vi "Ref_Num_Test_Conf.vi"(0 "Device Types":refnum<vi>, 1 "Test Fixtures":refnum<vi>, 2 "Test Signal Level":refnum<vi>, 4 "Device Type (OUTPUT)":refnum<vi>, 5 "Test Types":refnum<vi>, 6 "Test Fixture (OUTPUT)":refnum<vi>, 7 "Confirm Configuration":refnum<vi>, 10 "Test Type (OUTPUT)":refnum<vi>, 11 "error in":errorcluster, 12 "Category":refnum<vi>, 13 "LowCapMode?":refnum<vi>, 14 "CAPACITANCE TEST?":refnum<vi>) -> (15 "error out":errorcluster)   [LabVIEW 2020]
panel:
  in  "IGBT : Test Type":string[](array[string])
  in  "Transistor : Test Type":string[](array[string])
  in  "MOSFET : Test Type":string[](array[string])
  out "Fixture File Name":string
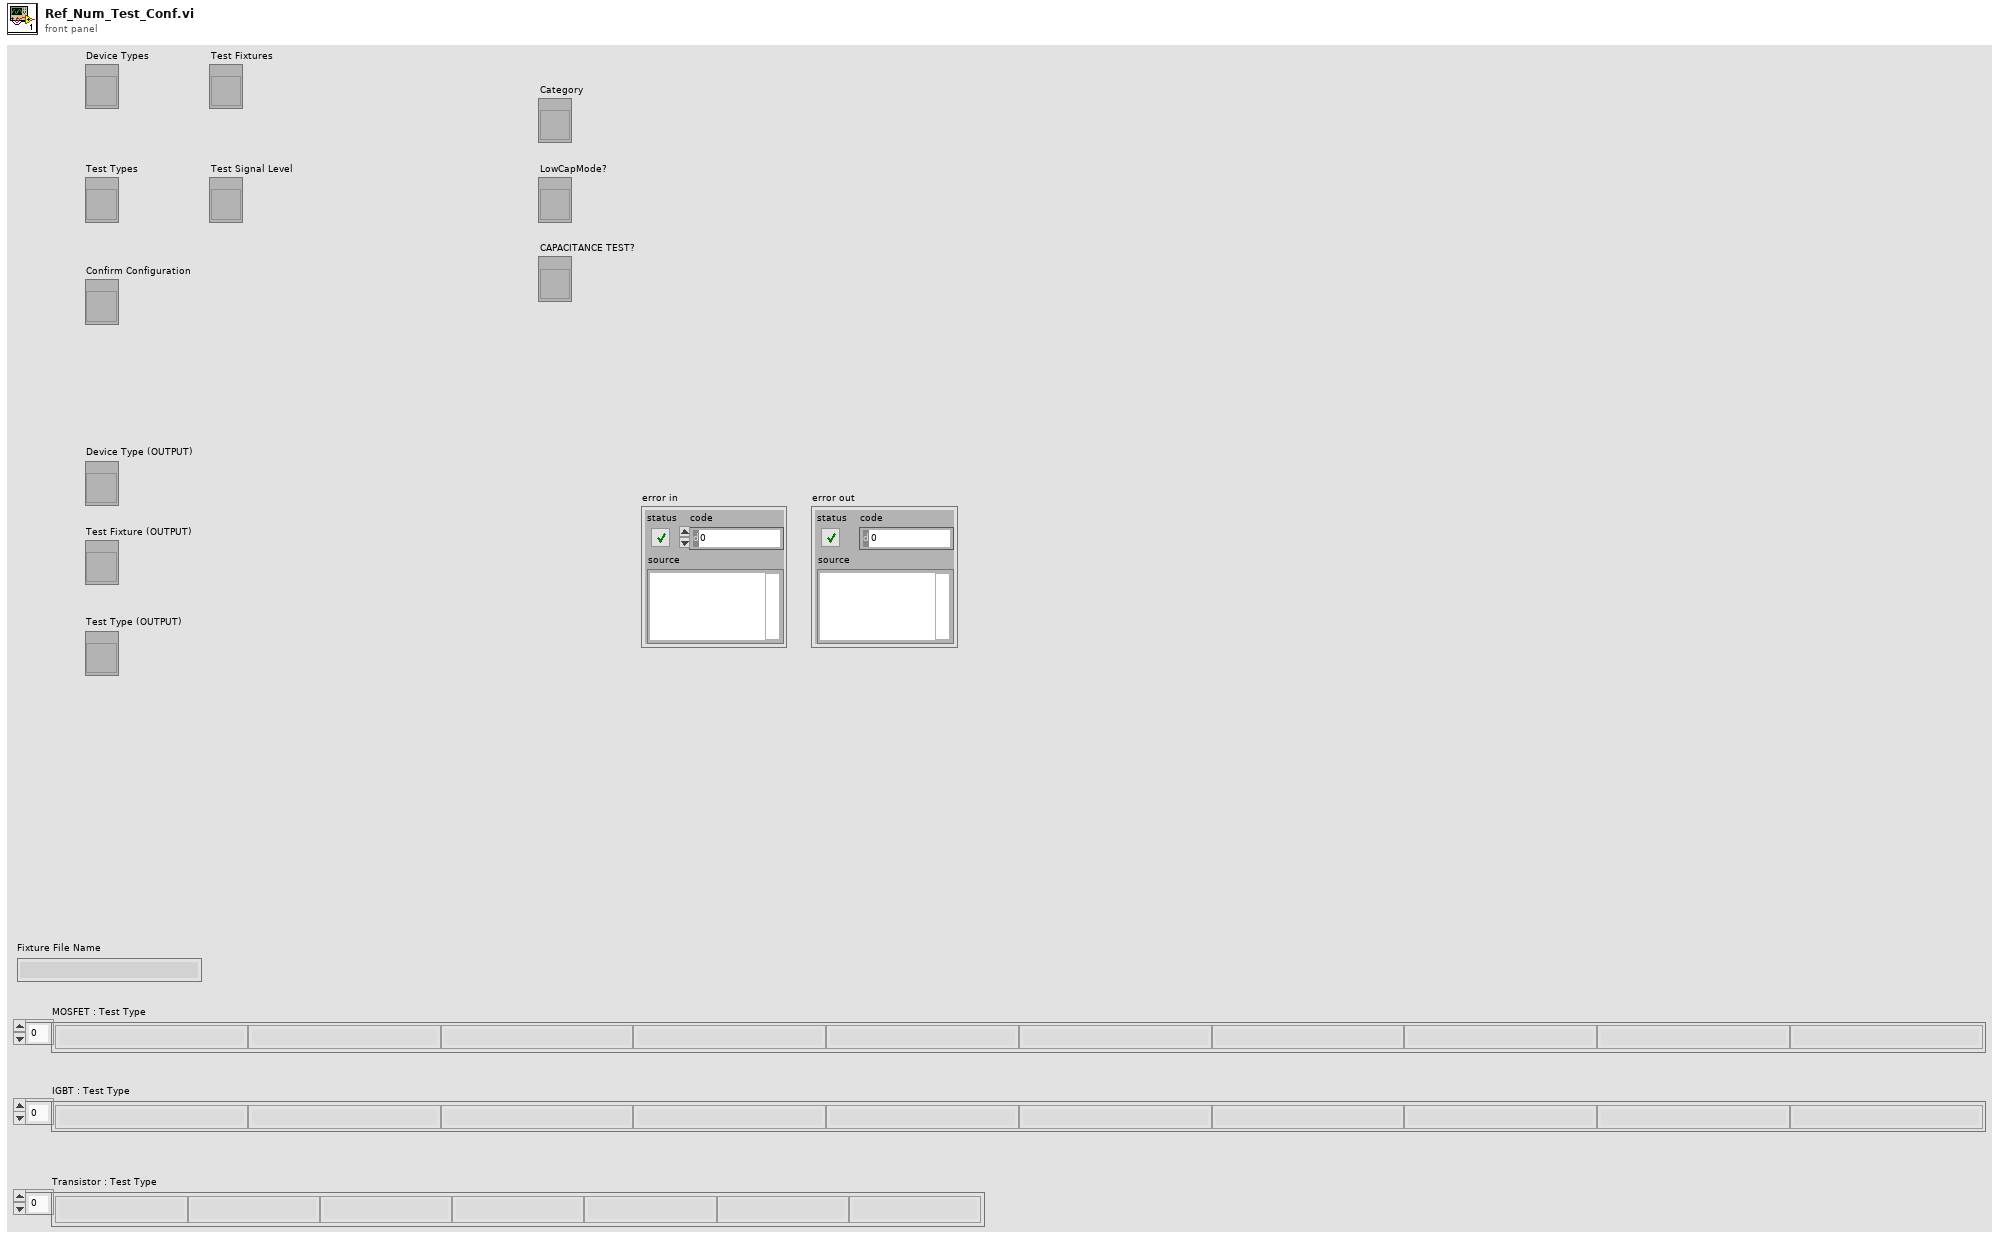
[diagram p1: front panel]
types:
  T1 = enum16{"Diode", "Transistor", "MOSFET", "Thyristor", "IGBT"}
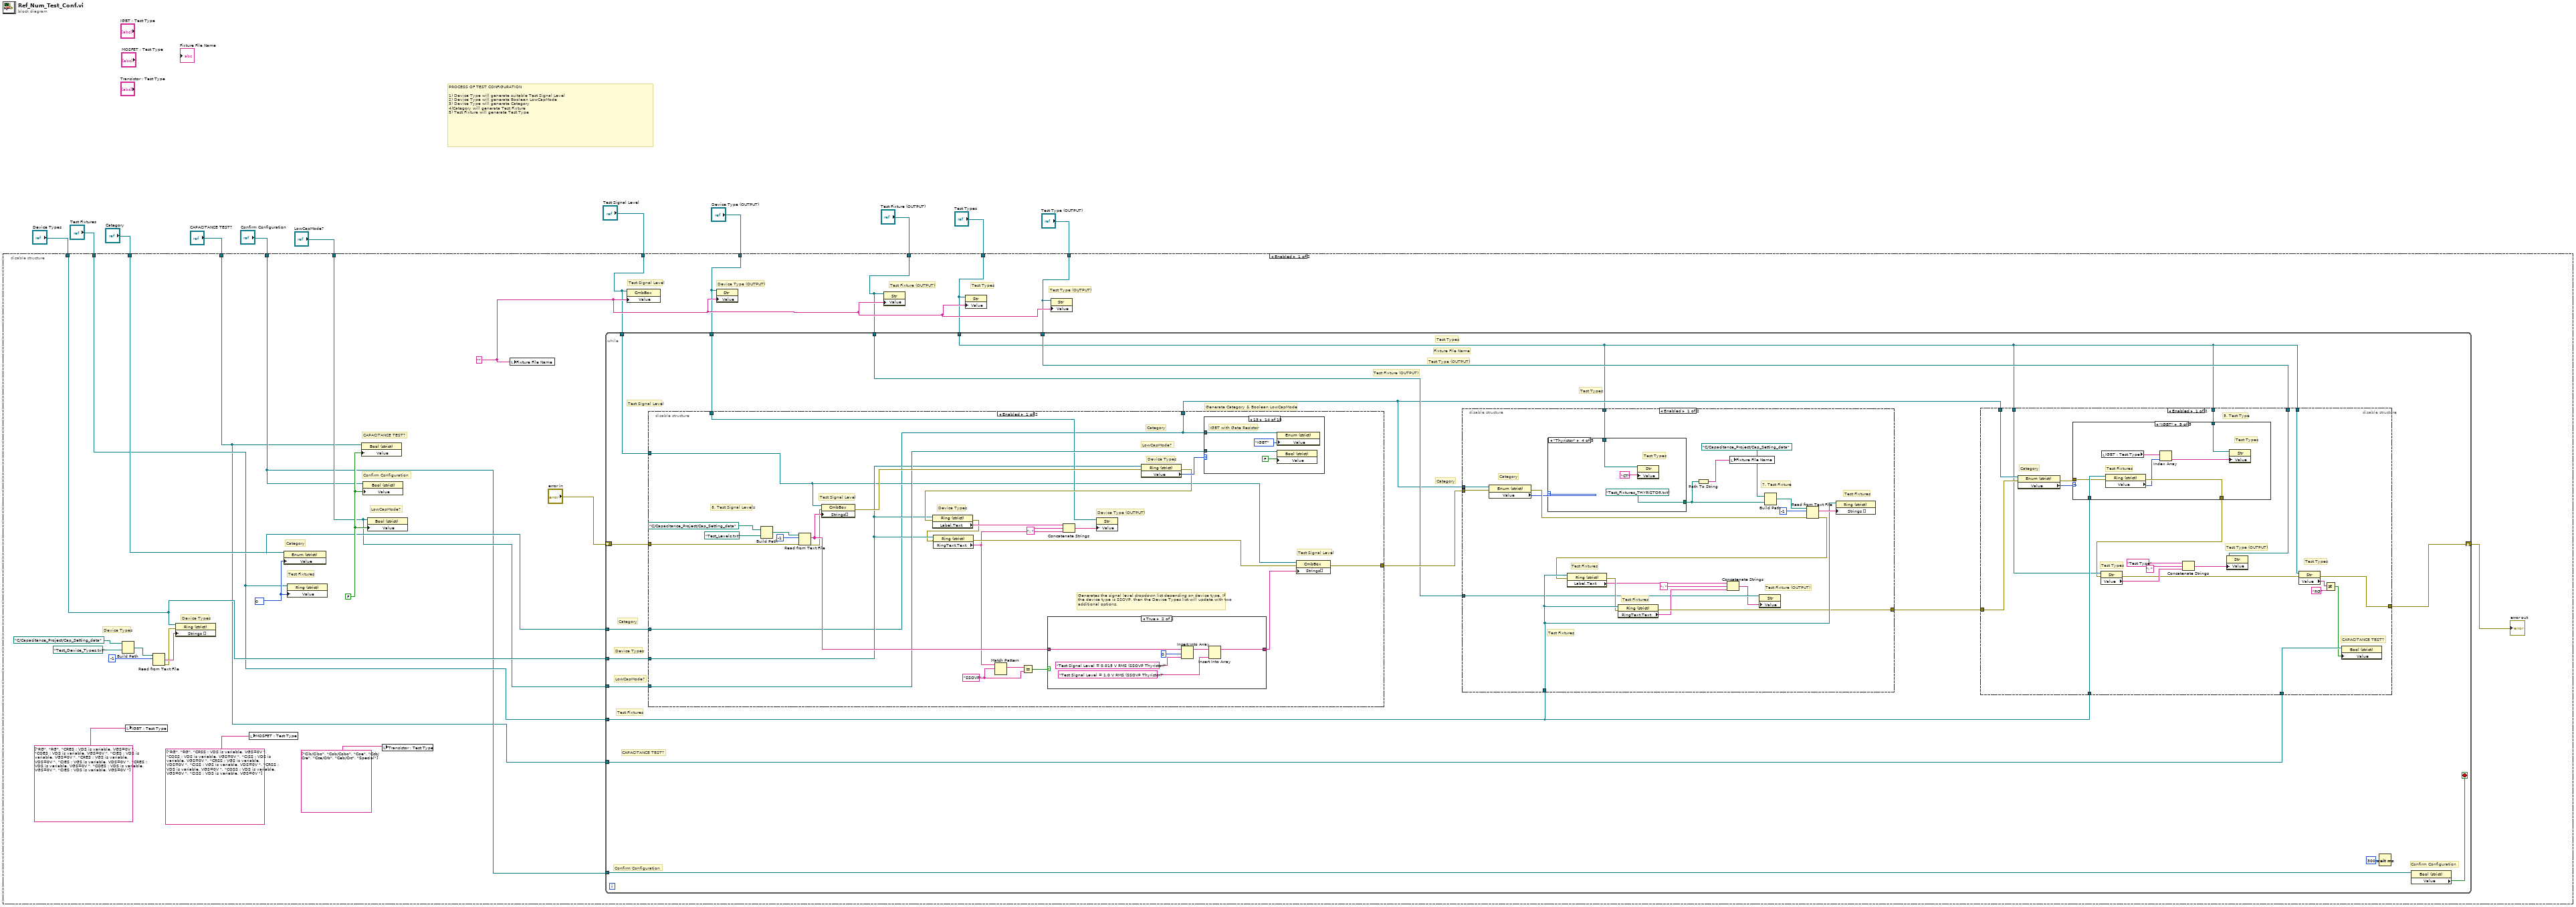
[diagram p0: block diagram]
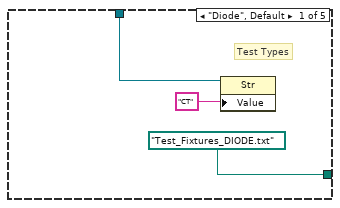
[diagram p2: hidden frame]
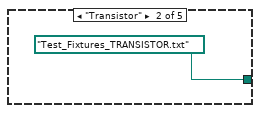
[diagram p3: hidden frame]
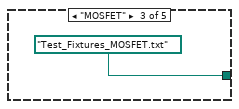
[diagram p4: hidden frame]
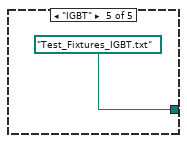
[diagram p5: hidden frame]
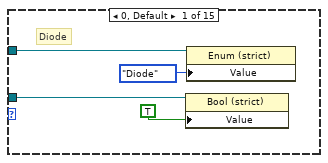
[diagram p7: hidden frame]
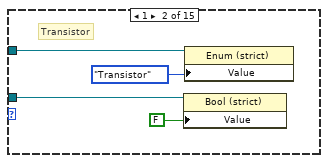
[diagram p8: hidden frame]
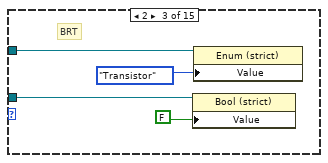
[diagram p9: hidden frame]
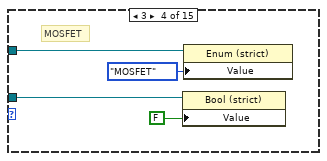
[diagram p10: hidden frame]
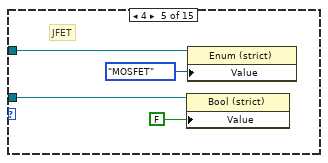
[diagram p11: hidden frame]
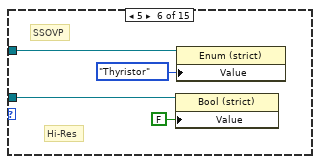
[diagram p12: hidden frame]
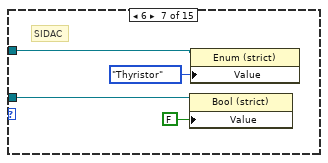
[diagram p13: hidden frame]
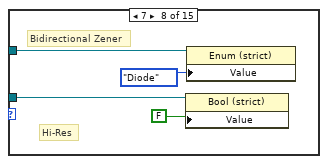
[diagram p14: hidden frame]
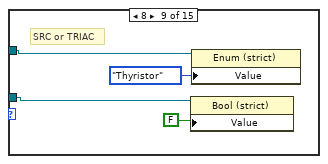
[diagram p15: hidden frame]
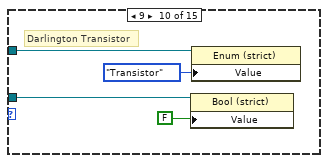
[diagram p16: hidden frame]
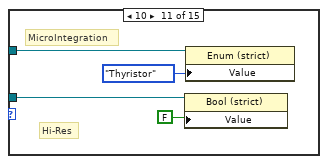
[diagram p17: hidden frame]
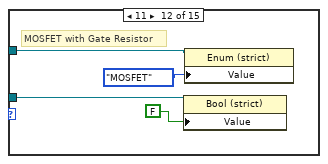
[diagram p18: hidden frame]
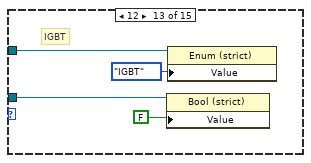
[diagram p19: hidden frame]
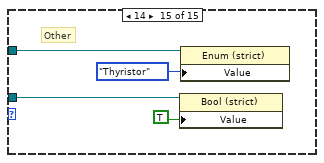
[diagram p20: hidden frame]
diagram:
  # "PROCESS OF TEST CONFIGURATION\n\n1) Device Type will generate suitable Test Signal Level\n2) Device Type will generate Boolean LowCapMode\n3) Device Type will generate Category\n4)Category will generate Test Fixture\n5) Test Fixture will generate Test Type"
  n1 = disable-structure shown="Enabled" {
    disable-tunnel: "Device Types" -> [w24 _]
    disable-tunnel: "Test Fixtures" -> [w19 _]
    disable-tunnel: "Category" -> [w23 _]
    disable-tunnel: "LowCapMode?" -> [w22 _]
    disable-tunnel: "Confirm Configuration" -> [w17 _]
    disable-tunnel: "CAPACITANCE TEST?" -> [w15 _]
    disable-tunnel: "Test Signal Level" -> [w25 _]
    disable-tunnel: "Device Type (OUTPUT)" -> [w21 _]
    disable-tunnel: "Test Fixture (OUTPUT)" -> [w18 _]
    disable-tunnel: "Test Types" -> [w20 _]
    disable-tunnel: "Test Type (OUTPUT)" -> [w16 _]
    frame Enabled {
      w28 = u16 0 items=[""]
      w27 = FALSE ("LowCapMode?")
      w26 = "" ("Category Check")
      # "Device Types"
      # "Test Type (OUTPUT)"
      # "Test Types"
      # "Test Fixture (OUTPUT)"
      # "Device Type (OUTPUT)"
      # "Test Signal Level"
      # "CAPACITANCE TEST?"
      # "Confirm Configuration"
      # "LowCapMode?"
      # "Category"
      # "Test Fixtures"
      # "Device Types"
      n2 = Build Path(base path=path "C:/Capacitance_Project/Cap_Setting_data", name or relative path=path "Test_Device_Types.txt" ("file (use dialog)")) -> (appended path=w36:path)
      n3 = local write "IGBT : Test Type"(string[] ["RG", "RG", "CRES : VDS is variable, VGS=0V ", "COES : VDS is variable, VGS=0V ", "CIES : VDS is variable, VGS=0V ", "CRES : VGS is variable, VDS=0V ", "CIES : VGS is variable, VDS=0V ", "CRES : VDS is variable, VGS=0V ", "COES : VDS is variable, VGS=0V ", "CIES : VDS is variable, VGS=0V "] ("MOSFET : Test Type")) -> ()
      n4 = Read from Text File(file (use dialog)=w36, count=-1) -> (text=w30:string[], error out=w29:errorcluster)  [unwired: 2 in, 2 out]
      n5 = property class="Ring (strict)"(reference=w24, error in=w29, "Strings []"=w30) -> ()  [unwired: 2 out]
      n6 = local write "MOSFET : Test Type"(string[] ["RG", "RG", "CRSS : VDS is variable, VGS=0V ", "COSS : VDS is variable, VGS=0V ", "CISS : VDS is variable, VGS=0V ", "CRSS : VGS is variable, VDS=0V ", "CISS : VGS is variable, VDS=0V ", "CRSS : VDS is variable, VGS=0V ", "COSS : VDS is variable, VGS=0V ", "CISS : VDS is variable, VGS=0V "] ("MOSFET : Test Type")) -> ()
      n7 = property class="Enum (strict)"(reference=w23, "Value"=w28) -> ()  [unwired: 1 in, 2 out]
      n8 = property class="Ring (strict)"(reference=w19, "Value"=w28) -> ()  [unwired: 1 in, 2 out]
      n9 = property class="Bool (strict)"(reference=w15, "Value"=w27) -> ()  [unwired: 1 in, 2 out]
      n10 = property class="Bool (strict)"(reference=w17, "Value"=w27) -> ()  [unwired: 1 in, 2 out]
      n11 = property class="Bool (strict)"(reference=w22, "Value"=w27) -> ()  [unwired: 1 in, 2 out]
      n12 = local write "Transistor : Test Type"(string[] ["Cib/Cibo", "Cob/Cobo", "Coe", "Ccb/Cre", "Cce/Crb", "Ceb/Crc", "Special"] ("IGBT : Test Type")) -> ()
      n13 = local write "Fixture File Name"(w26) -> ()
      n14 = while {
        shift-right: [w54] -> w14
        shift-left: "error in" -> [w53]
        tunnel: w25 -> [w50]
        tunnel: w24 -> [w49]
        tunnel: w23 -> [w48]
        tunnel: w22 -> [w47]
        tunnel: w21 -> [w46]
        tunnel: w20 -> [w38]
        tunnel: w19 -> [w40]
        tunnel: w18 -> [w44]
        tunnel: w17 -> [w42]
        tunnel: w16 -> [w39]
        tunnel: w15 -> [w37]
        stop <- w41 stop-if-true
        # "CAPACITANCE TEST?"
        # "Test Type (OUTPUT)"
        # "Confirm Configuration"
        # "Confirm Configuration"
        # "Category"
        # "Test Fixture (OUTPUT)"
        # "Test Fixtures"
        # "Fixture File Name"
        # "Test Types"
        # "Test Types"
        # "LowCapMode?"
        # "Generate Category & Boolean LowCapMode"
        # "Category"
        # "Device Types"
        # "Test Signal Level"
        n15 = disable-structure shown="Enabled" {
          disable-tunnel: [w88 _] -> w45
          disable-tunnel: w53 -> [w103 _]
          disable-tunnel: w50 -> [w91 _]
          disable-tunnel: w49 -> [w92 _]
          disable-tunnel: w48 -> [w85 _]
          disable-tunnel: w47 -> [w98 _]
          disable-tunnel: w46 -> [w94 _]
          disable-tunnel: [w85 _] -> w43
          frame Enabled {
            w108 = "SSOVP" ("regular expression")
            # "Test Signal Level"
            # "Device Type (OUTPUT)"
            # "Category"
            # "LowCapMode?"
            # "Device Types"
            # "Device Types"
            # "Test Signal Level"
            # "8. Test Signal Levels"
            # "Generates the signal level dropdown list depending on device type. If\nthe device type is SSOVP, then the Device Types list will update with two\nadditional options."
            n16 = Build Path(base path=path "C:/Capacitance_Project/Cap_Setting_data", name or relative path=path "Test_Levels.txt") -> (appended path=w106:path)
            n17 = Read from Text File(file (use dialog)=w106, count=-1, error in=w103) -> (text=w102:string[], error out=w101:errorcluster)  [unwired: 1 in, 2 out]
            n18 = property class="CmbBox"(reference=w91, error in=w101, "Strings[]"=w102) -> (error out=w100:errorcluster)  [unwired: 1 out]
            n19 = property class="Ring (strict)"(reference=w92, error in=w100) -> (error out=w97:errorcluster, "Value"=w99:u16)  [unwired: 1 out]
            n20 = property class="Ring (strict)"(reference=w92, error in=w97) -> (error out=w89:errorcluster, "Label.Text"=w95:string)  [unwired: 1 out]
            n21 = property class="Ring (strict)"(reference=w92, error in=w89) -> (error out=w90:errorcluster, "RingText.Text"=w86:string)  [unwired: 1 out]
            n22 = Match Pattern(string=w86, regular expression=w108) -> (match substring=w109:string)  [unwired: 1 in, 3 out]
            n23 = Equal?(x=w109, y=w108) -> (x = y?=w107:bool)
            n24 = case shown="True" w107 {
              tunnel: w102 -> [w170 w176]
              tunnel: [w170 w172] -> w87
              frame False {
              }
              frame True {
                n25 = Insert Into Array(array=w176, index=0, new element="Test Signal Level = 0.015 V RMS (SSOVP Thyristor)" ("new element/subarray")) -> (w173:string[])
                n26 = Insert Into Array(array=w173, new element="Test Signal Level = 1.0 V RMS (SSOVP Thyristor)" ("new element/subarray")) -> (w172:string[])  [unwired: 1 in]
              }
            }
            n27 = Concatenate Strings(w95, ": " ("string"), w86) -> (w93:string)
            n28 = property class="Str"(reference=w94, "Value"=w93) -> ()  [unwired: 1 in, 2 out]
            n29 = case shown="13" w99 {
              tunnel: w85 -> [w113 w117 w120 w125 w128 w133 w137 w141 w145 w149 w153 w157 w161 w165 w169]
              tunnel: w98 -> [w112 w115 w121 w124 w129 w132 w136 w140 w144 w148 w152 w156 w160 w164 w168]
              frame 0, Default {
                # "Diode"
                n30 = property class="Bool (strict)"(reference=w112, "Value"=TRUE ("LowCapMode?")) -> ()  [unwired: 1 in, 2 out]
                n31 = property class="Enum (strict)"(reference=w113, "Value"=T1."Diode" ("Category")) -> ()  [unwired: 1 in, 2 out]
              }
              frame 1 {
                # "Transistor"
                n32 = property class="Bool (strict)"(reference=w115, "Value"=FALSE ("LowCapMode?")) -> ()  [unwired: 1 in, 2 out]
                n33 = property class="Enum (strict)"(reference=w117, "Value"=T1."Transistor" ("Category")) -> ()  [unwired: 1 in, 2 out]
              }
              frame 2 {
                # "BRT"
                n34 = property class="Bool (strict)"(reference=w121, "Value"=FALSE ("LowCapMode?")) -> ()  [unwired: 1 in, 2 out]
                n35 = property class="Enum (strict)"(reference=w120, "Value"=T1."Transistor" ("Category")) -> ()  [unwired: 1 in, 2 out]
              }
              frame 3 {
                # "MOSFET"
                n36 = property class="Bool (strict)"(reference=w124, "Value"=FALSE ("LowCapMode?")) -> ()  [unwired: 1 in, 2 out]
                n37 = property class="Enum (strict)"(reference=w125, "Value"=T1."MOSFET" ("Category")) -> ()  [unwired: 1 in, 2 out]
              }
              frame 4 {
                # "JFET"
                n38 = property class="Bool (strict)"(reference=w129, "Value"=FALSE ("LowCapMode?")) -> ()  [unwired: 1 in, 2 out]
                n39 = property class="Enum (strict)"(reference=w128, "Value"=T1."MOSFET" ("Category")) -> ()  [unwired: 1 in, 2 out]
              }
              frame 5 {
                # "Hi-Res"
                # "SSOVP"
                n40 = property class="Bool (strict)"(reference=w132, "Value"=FALSE) -> ()  [unwired: 1 in, 2 out]
                n41 = property class="Enum (strict)"(reference=w133, "Value"=T1."Thyristor" ("Category")) -> ()  [unwired: 1 in, 2 out]
              }
              frame 6 {
                # "SIDAC"
                n42 = property class="Bool (strict)"(reference=w136, "Value"=FALSE ("LowCapMode?")) -> ()  [unwired: 1 in, 2 out]
                n43 = property class="Enum (strict)"(reference=w137, "Value"=T1."Thyristor" ("Category")) -> ()  [unwired: 1 in, 2 out]
              }
              frame 7 {
                # "Hi-Res"
                # "Bidirectional Zener"
                n44 = property class="Bool (strict)"(reference=w140, "Value"=FALSE ("LowCapMode?")) -> ()  [unwired: 1 in, 2 out]
                n45 = property class="Enum (strict)"(reference=w141, "Value"=T1."Diode" ("Category")) -> ()  [unwired: 1 in, 2 out]
              }
              frame 8 {
                # "SRC or TRIAC"
                n46 = property class="Bool (strict)"(reference=w144, "Value"=FALSE ("LowCapMode?")) -> ()  [unwired: 1 in, 2 out]
                n47 = property class="Enum (strict)"(reference=w145, "Value"=T1."Thyristor" ("Category")) -> ()  [unwired: 1 in, 2 out]
              }
              frame 9 {
                # "Darlington Transistor"
                n48 = property class="Bool (strict)"(reference=w148, "Value"=FALSE ("LowCapMode?")) -> ()  [unwired: 1 in, 2 out]
                n49 = property class="Enum (strict)"(reference=w149, "Value"=T1."Transistor" ("Category")) -> ()  [unwired: 1 in, 2 out]
              }
              frame 10 {
                # "Hi-Res"
                # "MicroIntegration"
                n50 = property class="Bool (strict)"(reference=w152, "Value"=FALSE ("LowCapMode?")) -> ()  [unwired: 1 in, 2 out]
                n51 = property class="Enum (strict)"(reference=w153, "Value"=T1."Thyristor" ("Category")) -> ()  [unwired: 1 in, 2 out]
              }
              frame 11 {
                # "MOSFET with Gate Resistor"
                n52 = property class="Bool (strict)"(reference=w156, "Value"=FALSE ("LowCapMode?")) -> ()  [unwired: 1 in, 2 out]
                n53 = property class="Enum (strict)"(reference=w157, "Value"=T1."MOSFET" ("Category")) -> ()  [unwired: 1 in, 2 out]
              }
              frame 12 {
                # "IGBT"
                n54 = property class="Bool (strict)"(reference=w160, "Value"=FALSE ("LowCapMode?")) -> ()  [unwired: 1 in, 2 out]
                n55 = property class="Enum (strict)"(reference=w161, "Value"=T1."IGBT" ("Category")) -> ()  [unwired: 1 in, 2 out]
              }
              frame 13 {
                # "IGBT with Gate Resistor"
                n56 = property class="Bool (strict)"(reference=w164, "Value"=FALSE ("LowCapMode?")) -> ()  [unwired: 1 in, 2 out]
                n57 = property class="Enum (strict)"(reference=w165, "Value"=T1."IGBT" ("Category")) -> ()  [unwired: 1 in, 2 out]
              }
              frame 14 {
                # "Other"
                n58 = property class="Bool (strict)"(reference=w168, "Value"=TRUE ("LowCapMode?")) -> ()  [unwired: 1 in, 2 out]
                n59 = property class="Enum (strict)"(reference=w169, "Value"=T1."Thyristor" ("Category")) -> ()  [unwired: 1 in, 2 out]
              }
            }
            n60 = property class="CmbBox"(reference=w91, error in=w90, "Strings[]"=w87) -> (error out=w88:errorcluster)  [unwired: 1 out]
          }
          frame Disabled {
          }
        }
        n61 = disable-structure shown="Enabled" {
          disable-tunnel: [w61 _] -> w52
          disable-tunnel: w43 -> [w70 _]
          disable-tunnel: w45 -> [w69 _]
          disable-tunnel: w38 -> [w66 _]
          disable-tunnel: w40 -> [w64 _]
          disable-tunnel: w44 -> [w58 _]
          frame Enabled {
            # "Test Fixture (OUTPUT)"
            # "Test Fixtures"
            # "Test Fixtures"
            # "Test Fixtures"
            # "Test Fixtures"
            # "7. Test Fixture"
            # "Category"
            n62 = property class="Enum (strict)"(reference=w70, error in=w69) -> (error out=w68:errorcluster, "Value"=w67:T1)  [unwired: 1 out]
            n63 = case shown="\"Thyristor\"" w67 {
              tunnel: [path "Test_Fixtures_DIODE.txt" ("file (use dialog)") path "Test_Fixtures_TRANSISTOR.txt" ("file (use dialog)") path "Test_Fixtures_MOSFET.txt" ("file (use dialog)") path "Test_Fixtures_THYRISTOR.txt" ("file (use dialog)") path "Test_Fixtures_IGBT.txt" ("file (use dialog)")] -> w71
              tunnel: w66 -> [w75 _ _ w81 _]
              frame "Diode", Default {
                # "Test Types"
                n64 = property class="Str"(reference=w75, "Value"="CT" ("Test Type")) -> ()  [unwired: 1 in, 2 out]
              }
              frame "Transistor" {
              }
              frame "MOSFET" {
              }
              frame "Thyristor" {
                # "Test Types"
                n65 = property class="Str"(reference=w81, "Value"="CT" ("Test Type")) -> ()  [unwired: 1 in, 2 out]
              }
              frame "IGBT" {
              }
            }
            n66 = Path To String(path=w71) -> (string=w56:string)
            n67 = local write "Fixture File Name"(w56) -> ()
            n68 = Build Path(base path=path "C:/Capacitance_Project/Cap_Setting_data", name or relative path=w71) -> (appended path=w72:path)
            n69 = Read from Text File(file (use dialog)=w72, count=-1, error in=w68) -> (text=w65:string[], error out=w63:errorcluster)  [unwired: 1 in, 2 out]
            n70 = property class="Ring (strict)"(reference=w64, error in=w63) -> (error out=w62:errorcluster, "Label.Text"=w60:string)  [unwired: 1 out]
            n71 = property class="Ring (strict)"(reference=w64, error in=w62) -> (error out=w61:errorcluster, "RingText.Text"=w59:string)  [unwired: 1 out]
            n72 = Concatenate Strings(w60, ": " ("string"), w59) -> (w57:string)
            n73 = property class="Str"(reference=w58, "Value"=w57) -> ()  [unwired: 1 in, 2 out]
            n74 = property class="Ring (strict)"(reference=w64, "Strings []"=w65) -> ()  [unwired: 1 in, 2 out]
          }
          frame Disabled {
          }
        }
        n75 = disable-structure shown="Enabled" {
          disable-tunnel: w52 -> [w192 _]
          disable-tunnel: [w181 _] -> w54
          disable-tunnel: w43 -> [w193 _]
          disable-tunnel: w38 -> [w189 _]
          disable-tunnel: w40 -> [w188 _]
          disable-tunnel: w38 -> [w187 _]
          disable-tunnel: w39 -> [w184 _]
          disable-tunnel: w38 -> [w180 _]
          disable-tunnel: w37 -> [w178 _]
          frame Enabled {
            # "CAPACITANCE TEST?"
            # "Test Types"
            # "Test Type (OUTPUT)"
            # "Test Types"
            # "Category"
            # "5. Test Type"
            n76 = property class="Enum (strict)"(reference=w193, error in=w192) -> (error out=w190:errorcluster, "Value"=w191:T1)  [unwired: 1 out]
            n77 = case shown="\"IGBT\"" w191 {
              tunnel: w190 -> [w199 w203 w209 w216 w219]
              tunnel: [w199 w202 w208 w216 w218] -> w186
              tunnel: w189 -> [w198 w206 w211 w215 w223]
              tunnel: w188 -> [_ w200 w210 _ w220]
              frame "Diode", Default {
                # "Test Types"
                n78 = property class="Str"(reference=w198, "Value"="CT" ("Test Type")) -> ()  [unwired: 1 in, 2 out]
              }
              frame "Transistor" {
                # "Test Fixtures"
                # "Test Types"
                n79 = local read "Transistor : Test Type"() -> (w204:string[])
                n80 = property class="Ring (strict)"(reference=w200, error in=w203) -> (error out=w202:errorcluster, "Value"=w201:u16)  [unwired: 1 out]
                n81 = Index Array(array=w204, index=w201) -> (element=w205:string)
                n82 = property class="Str"(reference=w206, "Value"=w205) -> ()  [unwired: 1 in, 2 out]
              }
              frame "MOSFET" {
                # "Test Fixtures"
                # "Test Types"
                n83 = property class="Ring (strict)"(reference=w210, error in=w209) -> (error out=w208:errorcluster, "Value"=w207:u16)  [unwired: 1 out]
                n84 = local read "MOSFET : Test Type"() -> (w213:string[])
                n85 = Index Array(array=w213, index=w207) -> (element=w212:string)
                n86 = property class="Str"(reference=w211, "Value"=w212) -> ()  [unwired: 1 in, 2 out]
              }
              frame "Thyristor" {
                # "Test Types"
                n87 = property class="Str"(reference=w215, "Value"="CT" ("Test Type")) -> ()  [unwired: 1 in, 2 out]
              }
              frame "IGBT" {
                # "Test Fixtures"
                # "Test Types"
                n88 = local read "IGBT : Test Type"() -> (w221:string[])
                n89 = property class="Ring (strict)"(reference=w220, error in=w219) -> (error out=w218:errorcluster, "Value"=w217:u16)  [unwired: 1 out]
                n90 = Index Array(array=w221, index=w217) -> (element=w222:string)
                n91 = property class="Str"(reference=w223, "Value"=w222) -> ()  [unwired: 1 in, 2 out]
              }
            }
            n92 = property class="Str"(reference=w187, error in=w186) -> (error out=w182:errorcluster, "Value"=w185:string)  [unwired: 1 out]
            n93 = Concatenate Strings("Test Type" ("string"), ": " ("string"), w185) -> (w183:string)
            n94 = property class="Str"(reference=w184, "Value"=w183) -> ()  [unwired: 1 in, 2 out]
            n95 = property class="Str"(reference=w180, error in=w182) -> (error out=w181:errorcluster, "Value"=w179:string)  [unwired: 1 out]
            n96 = Not Equal?(x=w179, y="RG") -> (x != y?=w177:bool)
            n97 = property class="Bool (strict)"(reference=w178, "Value"=w177) -> ()  [unwired: 1 in, 2 out]
          }
          frame Disabled {
          }
        }
        n98 = Wait (ms)(milliseconds to wait=u32 300) -> ()  [unwired: 1 out]
        n99 = property class="Bool (strict)"(reference=w42) -> ("Value"=w41:bool)  [unwired: 1 in, 2 out]
      }
      "error out" <- w14
      n100 = property class="CmbBox"(reference=w25, "Value"=w26) -> ()  [unwired: 1 in, 2 out]
      n101 = property class="Str"(reference=w21, "Value"=w26) -> ()  [unwired: 1 in, 2 out]
      n102 = property class="Str"(reference=w18, "Value"=w26) -> ()  [unwired: 1 in, 2 out]
      n103 = property class="Str"(reference=w20, "Value"=w26) -> ()  [unwired: 1 in, 2 out]
      n104 = property class="Str"(reference=w16, "Value"=w26) -> ()  [unwired: 1 in, 2 out]
    }
    frame Disabled {
    }
  }
